vi "Set Plugin.vi"(7 "error in (no error)":errorcluster, 8 "plugin index":i32, 9 "plugin config":T1={"name"="Plugin", "components"=[], "cycle timing"={"priority"=10000, "decimation"=1, "offset"=0}, "threads"=[], "transfer groups"=[], "settings"=[]} {"transfer groups"."transfers"."channels"."string offset" format="%d bytes"}, 10 "configuration session in":refnum<class "Configuration Session.lvclass">) -> (0 "error out":errorcluster, 1 "replaced existing?":bool, 3 "configuration session out":refnum<class "Configuration Session.lvclass">)   [LabVIEW 2017, in "DSF Core.lvlib" / "Configuration Session.lvclass"]
doc: "Determines whether a configuration data dsf refnum is valid."
uses:
  Configuration Session.lvclass
  Typedefs/DSF Engine Plugin Configuration.ctl
  Typedefs/DSF Timing Info.ctl
  Typedefs/DSF Engine Plugin Thread Configuration.ctl
  Typedefs/DSF Settings Info.ctl
  Typedefs/DSF Engine Transfer Group Configuration.ctl
  Typedefs/DSF Direction.ctl
  Typedefs/DSF Engine Transfer Configuration.ctl
  Typedefs/DSF Byte Order.ctl
  Typedefs/DSF Engine Channel Configuration.ctl
  Typedefs/DSF Data Type.ctl
  Typedefs/DSF Timeout Behavior.ctl
  Configuration Session.lvclass/Configuration Session.ctl
  DSF Core.lvlib
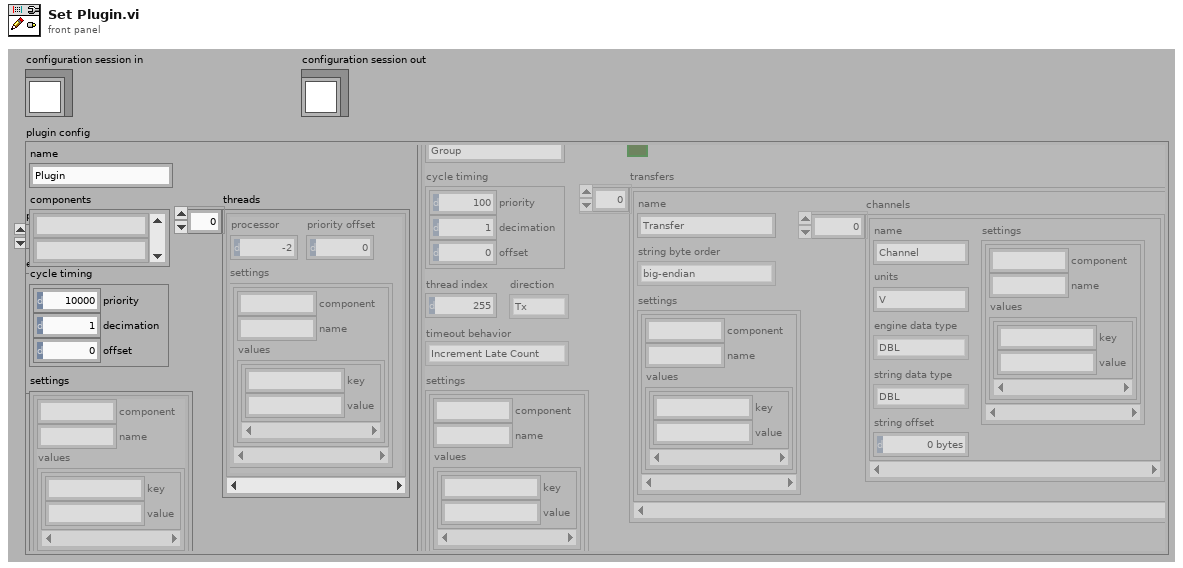
[diagram p1: front panel]
types:
  T1 = typedef "DSF Core.lvlib/DSF Engine Plugin Configuration.ctl" = cluster{"name":string, "components":string[], "cycle timing":T2, "threads":T3[], "transfer groups":T5[], "settings":T4}
  T2 = typedef "DSF Core.lvlib/DSF Timing Info.ctl" = cluster{"priority":u64, "decimation":u64, "offset":u64}
  T3 = typedef "DSF Core.lvlib/DSF Engine Plugin Thread Configuration.ctl" = cluster{"processor":i32, "priority offset":i16, "settings":T4}
  T4 = typedef "DSF Core.lvlib/DSF Settings Info.ctl" = cluster{"component":string, "name":string, "values":cluster{"key":string, "value":string}[]}[]
  T5 = typedef "DSF Core.lvlib/DSF Engine Transfer Group Configuration.ctl" = cluster{"name":string, "direction":T6, "cycle timing":T2, "thread index":u8, "settings":T4, "transfers":T7[], "timeout behavior":T11, "convert buffers":bool}
  T6 = typedef "DSF Core.lvlib/DSF Direction.ctl" = enum8{"Tx", "Rx"}
  T7 = typedef "DSF Core.lvlib/DSF Engine Transfer Configuration.ctl" = cluster{"name":string, "string byte order":T8, "settings":T4, "channels":T9[]}
  T8 = typedef "DSF Core.lvlib/DSF Byte Order.ctl" = enum8{"big-endian", "little-endian"}
  T9 = typedef "DSF Core.lvlib/DSF Engine Channel Configuration.ctl" = cluster{"string offset":u64, "name":string, "units":string, "engine data type":T10, "string data type":T10, "settings":T4}
  T10 = typedef "DSF Core.lvlib/DSF Data Type.ctl" = enum8{"Bool", "SGL", "DBL", "I8", "I16", "I32", "I64", "U8", "U16", "U32", "U64"}
  T11 = typedef "DSF Core.lvlib/DSF Timeout Behavior.ctl" = enum8{"Increment Late Count", "Throw Error"}
  T12 = typedef "DSF Core.lvlib/Configuration Session.lvclass/DSF Config Data Ref.ctl" = refnum<data-value>
  T13 = typedef "DSF Core.lvlib/Configuration Session.lvclass/DSF Config Data.ctl" = cluster{"dsf configuration":T14, "path":path, "dirty":bool}
  T14 = typedef "DSF Core.lvlib/Configuration Session.lvclass/Internal DSF Configuration.ctl" = cluster{"dsfversion":T15, "version":T15, "plugins":T16[], "groups":T18[], "transfers":T20[], "channels":T22[], "settings":T24[], "framework configuration":T26}
  T15 = typedef "DSF Core.lvlib/DSF Version Info.ctl" = cluster{"major":u32, "minor":u32, "fix":u32, "build":string}
  T16 = typedef "DSF Core.lvlib/Configuration Session.lvclass/Internal DSF Plugin with ID.ctl" = cluster{"id":string, "values":T17}
  T17 = typedef "DSF Core.lvlib/Configuration Session.lvclass/Internal DSF Plugin Info.ctl" = cluster{"components":string[], "timing":T2, "group ids":string[], "settings id":string, "threads":T3[]}
  T18 = typedef "DSF Core.lvlib/Configuration Session.lvclass/Internal DSF Group with ID.ctl" = cluster{"id":string, "values":T19}
  T19 = typedef "DSF Core.lvlib/Configuration Session.lvclass/Internal DSF Group Info.ctl" = cluster{"direction":i32, "timing":T2, "transfer ids":string[], "settings id":string, "thread":i32, "timeout behavior":u8}
  T20 = typedef "DSF Core.lvlib/Configuration Session.lvclass/Internal DSF Transfer with ID.ctl" = cluster{"id":string, "values":T21}
  T21 = typedef "DSF Core.lvlib/Configuration Session.lvclass/Internal DSF Transfer Info.ctl" = cluster{"byte order":i32, "channel ids":string[], "settings id":string}
  T22 = typedef "DSF Core.lvlib/Configuration Session.lvclass/Internal DSF Channel with ID.ctl" = cluster{"id":string, "values":T23}
  T23 = typedef "DSF Core.lvlib/Configuration Session.lvclass/Internal DSF Channel Info.ctl" = cluster{"string buffer offset":u64, "string data type":i32, "engine data type":i32, "settings id":string, "units":string}
  T24 = typedef "DSF Core.lvlib/Configuration Session.lvclass/Internal DSF Settings with ID.ctl" = cluster{"id":string, "values":T25}
  T25 = typedef "DSF Core.lvlib/Configuration Session.lvclass/Internal DSF Settings Info.ctl" = cluster{"key":string, "value":string}[]
  T26 = typedef "DSF Core.lvlib/DSF Engine Framework Configuration.ctl" = cluster{"plugins":T1[]}
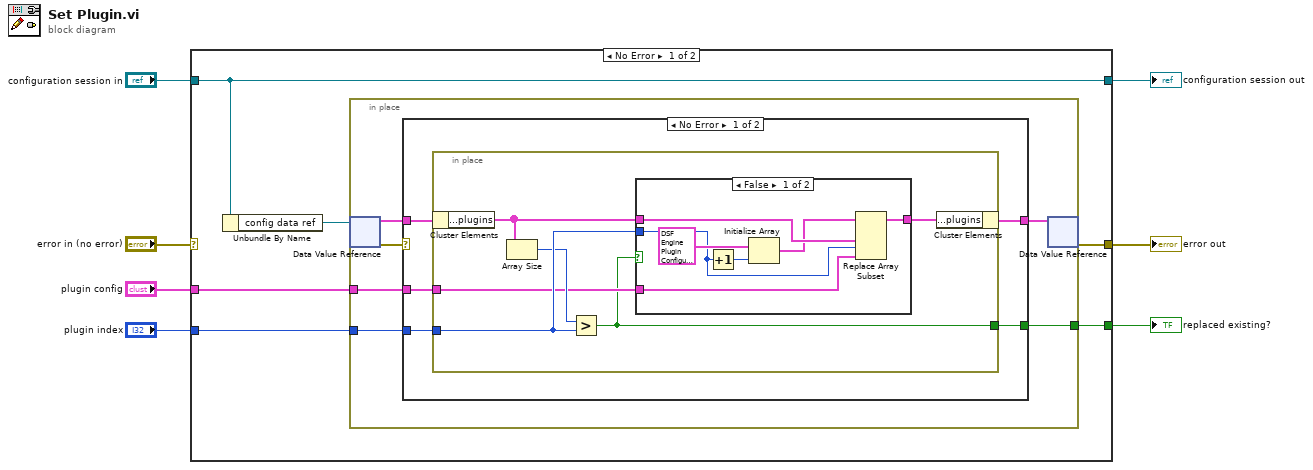
[diagram p0: block diagram]
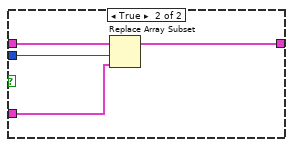
[diagram p2: hidden frame]
diagram:
  n1 = case shown="No Error" "error in (no error)" {
    selector: "error in (no error)" -> [_ w44]
    tunnel: [w13 w44] -> w7
    tunnel: "plugin config" -> [w12 _]
    tunnel: "configuration session in" -> [w10 w43]
    tunnel: [w10 w43] -> w4
    tunnel: "plugin index" -> [w9 _]
    tunnel: [w8 _] -> w1
    frame No Error {
      n2 = Unbundle By Name(w10) -> ("config data ref"=w11:T12)
      n3 = in-place {
        in-place-border: w12 -> [w18]
        in-place-border: w9 -> [w15]
        in-place-border: [w14] -> w8
        n4 = in-place-dvr #1(w11) -> (w19:T13, w17:errorcluster)
        n5 = case shown="No Error" w17 {
          tunnel: w19 -> [w24 w42]
          tunnel: w18 -> [w23 _]
          tunnel: [w22 w42] -> w16
          tunnel: w15 -> [w21 _]
          tunnel: [w20 _] -> w14
          frame No Error {
            n6 = in-place {
              in-place-border: w23 -> [w27]
              in-place-border: w21 -> [w29]
              in-place-border: [w25] -> w20
              n7 = in-place-cluster #2(w24) -> ("dsf configuration.framework configuration.plugins"=w30:T1[])
              n8 = Array Size(array=w30) -> (size(s)=w28:i32)
              n9 = Greater?(x=w28, y=w29) -> (0:w25:bool)
              n10 = case shown="False" w25 {
                tunnel: w30 -> [w35 w41]
                tunnel: w29 -> [w32 w40]
                tunnel: w27 -> [w31 w39]
                tunnel: [w34 w38] -> w26
                frame False {
                  n11 = Increment(x=w32) -> (x+1=w37:i32)
                  n12 = Initialize Array(T1 {"name"="Plugin", "components"=[], "cycle timing"={"priority"=10000, "decimation"=1, "offset"=0}, "threads"=[], "transfer groups"=[], "settings"=[]} ("plugin config"), w37) -> (w33:T1[])
                  n13 = Replace Array Subset(array=w33, new element #1=w35, new element #2=w31, index #2=w32) -> (w34:T1[])  [unwired: 1 in]
                }
                frame True {
                  n14 = Replace Array Subset(array=w41, new element=w39, index=w40) -> (w38:T1[])
                }
              }
              n15 = in-place-cluster #2("dsf configuration.framework configuration.plugins"=w26) -> (w22:T13)
            }
          }
          frame Error {
          }
        }
        n16 = in-place-dvr #1(w16) -> (w13:errorcluster)  [unwired: 1 out]
      }
    }
    frame Error {
    }
  }
  "configuration session out" <- w4
  "error out" <- w7
  "replaced existing?" <- w1
